vi "Target Logger State Manager.vi"(8 "Valid for Logging?":bool, 11 "Previous State":T2=enum."Accumulate") -> (3 "Current State":T1(ring)=enum."Accumulate", 6 "Preallocate Array?":bool)   [LabVIEW 2018]
uses:
  Target Logger States.ctl
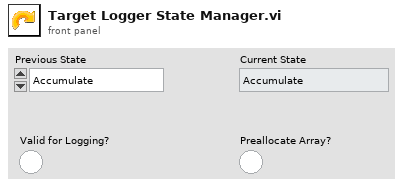
[diagram p1: front panel]
types:
  T1 = enum16{"Idle", "Accumulate", "Write Main", "Write Metadata"}
  T2 = typedef "Target Logger States.ctl" = enum16{"Idle", "Accumulate", "Write Main", "Write Metadata"}
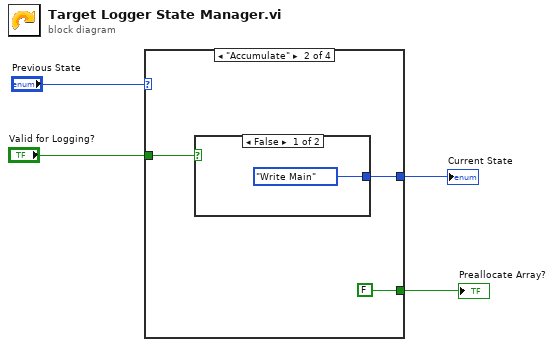
[diagram p0: block diagram]
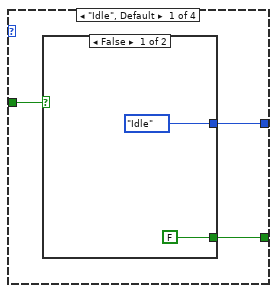
[diagram p2: hidden frame]
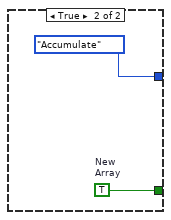
[diagram p3: hidden frame]
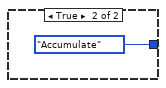
[diagram p4: hidden frame]
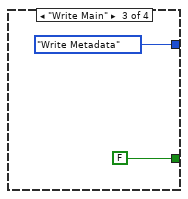
[diagram p5: hidden frame]
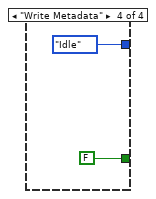
[diagram p6: hidden frame]
diagram:
  n1 = case shown="\"Accumulate\"" "Previous State" {
    tunnel: "Valid for Logging?" -> [w7 w14 _ _]
    tunnel: [w6 w13 Target_Logger_States."Write Metadata" ("Enum") Target_Logger_States."Idle" ("Enum")] -> w2
    tunnel: [w5 FALSE ("New\nArray") FALSE ("New\nArray") FALSE ("New\nArray")] -> w1
    frame "Idle", Default {
      n2 = case shown="False" w7 {
        tunnel: [Target_Logger_States."Idle" ("Enum") Target_Logger_States."Accumulate"] -> w6
        tunnel: [FALSE w10] -> w5
        frame False {
        }
        frame True {
          w10 = TRUE  # New Array
        }
      }
    }
    frame "Accumulate" {
      n3 = case shown="False" w14 {
        tunnel: [Target_Logger_States."Write Main" ("Enum") Target_Logger_States."Accumulate" ("Enum")] -> w13
        frame False {
        }
        frame True {
        }
      }
    }
    frame "Write Main" {
    }
    frame "Write Metadata" {
    }
  }
  "Current State" <- w2
  "Preallocate Array?" <- w1
